vi "Get New Incrementing File Object.vi"(8 "error in":errorcluster, 10 "Condition":bool, 11 "File Splitting Logger in":refnum<class "File Splitting Logger.lvclass">) -> (0 "error out":errorcluster, 3 "File Splitting Logger out":refnum<class "File Splitting Logger.lvclass">)   [LabVIEW 2020, in "File Splitting Logger.lvclass"]
uses:
  File Splitting Logger.lvclass
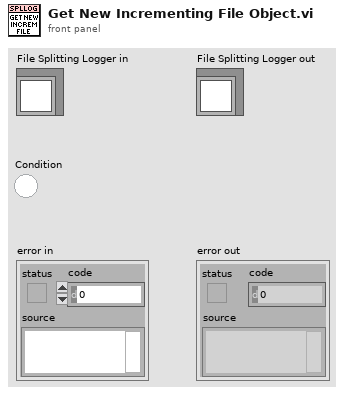
[diagram p1: front panel]
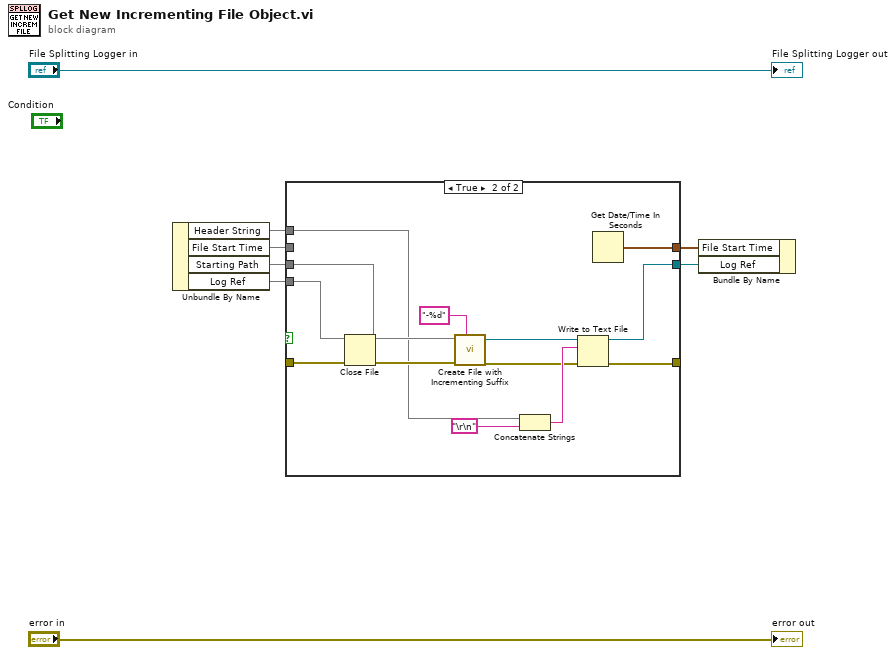
[diagram p0: block diagram]
diagram:
  n1 = Unbundle By Name() -> ("Header String"=w1, "File Start Time"=w3, "Starting Path"=w2, "Log Ref"=w6)  [unwired: 1 in]
  n2 = case shown="True" w5 {
    tunnel: w6 -> [w13 w25]
    tunnel: [w13 w15] -> w7
    tunnel: [w12 w23] -> w8
    tunnel: [w12 w14] -> _
    tunnel: [w11 w22] -> w4
    tunnel: w3 -> [w11 _]
    tunnel: w2 -> [_ w21]
    tunnel: w1 -> [_ w18]
    frame False {
    }
    frame True {
      n3 = Close File(refnum=w25, error in=w23) -> (error out=w24:errorcluster)  [unwired: 1 out]
      n4 = call <vilib>:"Create File with Incrementing Suffix.vi"("format string (\" (%d)\")"="-%d" ("format string (\" (%d)\")"), "error in (no error)"=w24, "file path"=w21) -> ("error out"=w16:errorcluster, "refnum out"=w17:refnum<file>)  [unwired: 6 in, 1 out]
      n5 = Concatenate Strings(w18, "\r\n") -> (w20:string)
      n6 = Write to Text File(file (use dialog)=w17, text=w20, error in=w16) -> (refnum out=w15:refnum<file>, error out=w14:errorcluster)  [unwired: 1 in, 1 out]
      n7 = Get Date/Time In Seconds() -> (seconds since 1Jan1904=w22:timestamp)
    }
  }
  n8 = Bundle By Name("File Start Time"=w4, "Log Ref"=w7) -> ()  [unwired: 1 in, 1 out]
  "error out" <- "error in"
  "File Splitting Logger out" <- "File Splitting Logger in"
